vi "On Click Show Calibration Board.vi"(8 "error in (no error)":errorcluster, 11 "App in":refnum<class "App.lvclass">) -> (0 "error out":errorcluster, 3 "App out":refnum<class "App.lvclass">)   [LabVIEW 2020, in "AR Example.lvlib" / "App.lvclass"]
uses:
  App.lvclass
  App.lvclass/App.ctl
  UI/UI.lvclass
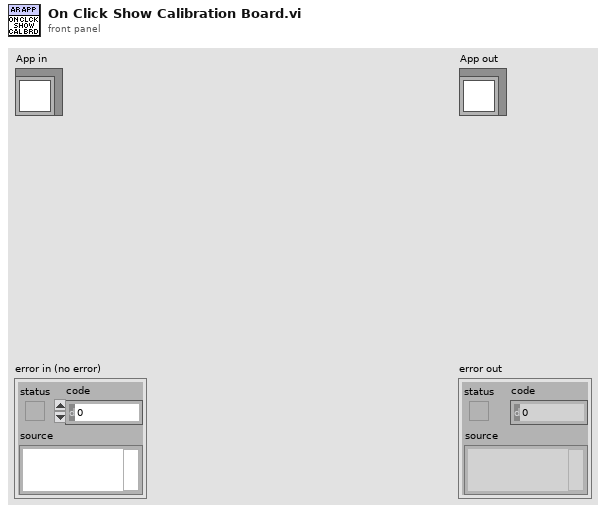
[diagram p1: front panel]
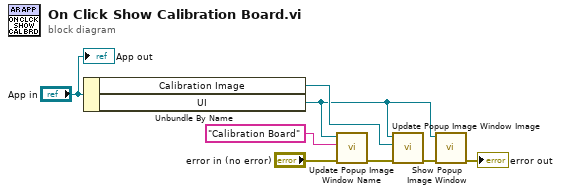
[diagram p0: block diagram]
diagram:
  n1 = Unbundle By Name("App in") -> ("Calibration Image"=w5:refnum<data-value>, "UI"=w3:refnum<class "UI.lvclass">)
  n2 = call "Update Popup Image Window Name.vi"("error in (no error)"="error in (no error)", "Window Name"="Calibration Board", "UI in"=w3) -> ("error out"=w4:errorcluster)  [unwired: 8 in]
  n3 = call "Update Popup Image Window Image.vi"("error in (no error)"=w4, "Image"=w5, "UI in"=w3) -> ("error out"=w2:errorcluster)  [unwired: 8 in]
  n4 = call "Show Popup Image Window.vi"("error in (no error)"=w2, "UI in"=w3) -> ("error out"=→"error out":errorcluster)  [unwired: 9 in]
  "App out" <- "App in"
